vi "DIAdem Request Query.vi"(5 "Logic String":string, 6 "result columns (comma list)":string, 7 "Conditions String":string, 8 "error in (no error)":errorcluster, 9 "Username (empty)":string, 10 "Query Name":string="Spartan_Query.VBS", 11 "Query TDM":path) -> (0 "error out":errorcluster, 2 "Timed Out?":bool, 3 "Result":string)   [LabVIEW 2011]
uses:
  DIAdem Daemon Queue.ctl
  DIAdem Daemon Script Type.ctl
  Addons/internet/utils/strutil.llb/Case Matching.ctl
  server lib/Spartan CONFIG Global.vi
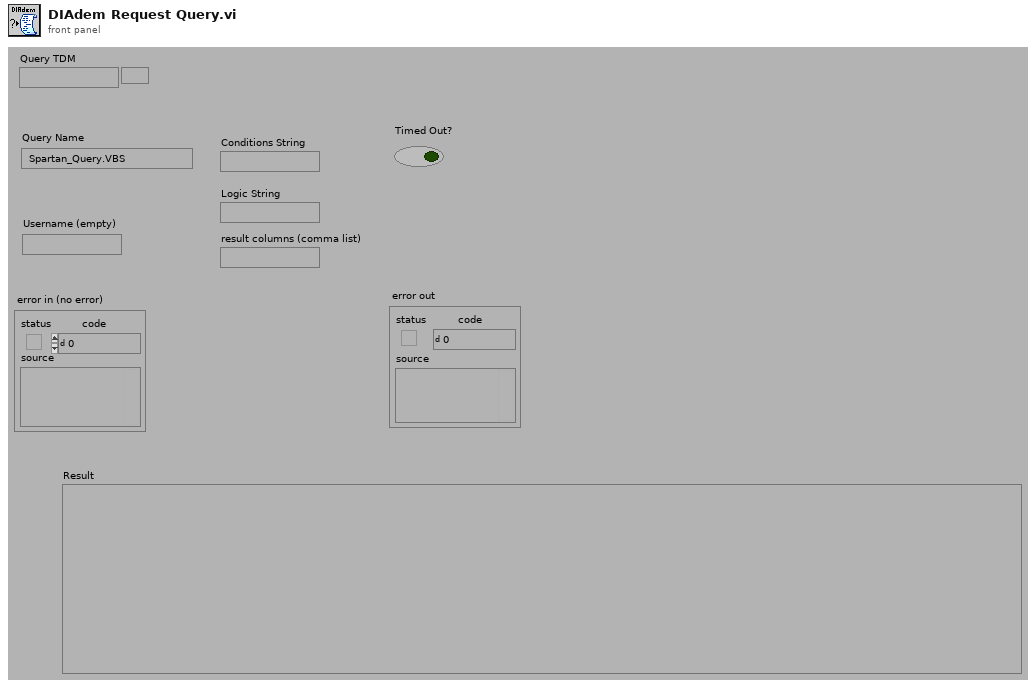
[diagram p1: front panel]
types:
  T1 = typedef "Case Matching.ctl" = enum16{"a != A", "a == A", "system"}
  T2 = typedef "DIAdem Daemon Script Type.ctl" = enum16{"Report", "Query", "Script", "Datasheet", "Append", "Restart", "Stop"}
  T3 = typedef "DIAdem Daemon Queue.ctl" = cluster{"Report Template TDM":path, "Report Processor VBS":path, "Report Path PDF":path, "Report Script Params":string, "Username":string, "Script Type":T2, "Report Query Params":string, "Client Machine":string, "Print on Client?":bool, "Response Queue Name":string, "Script Variables":string[], "Start Request Time":timestamp, "Wait?":bool}
  T4 = typedef "Keyed Array.ctl" = cluster{"keys":string[], "values":string[]}
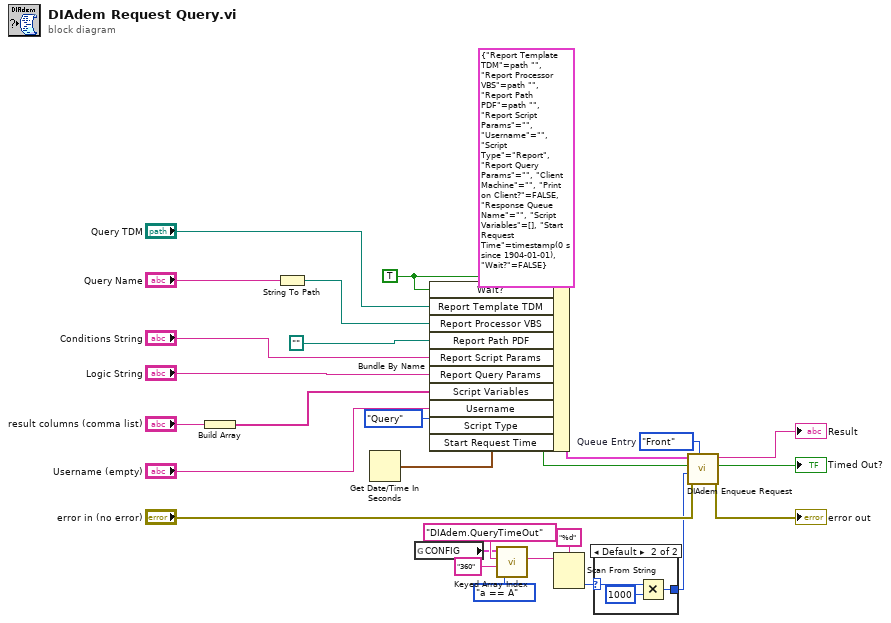
[diagram p0: block diagram]
diagram:
  w12 = enum16{"Front", "Back"}."Front"  # Queue Entry
  w9 = TRUE ("Wait for Completion?")
  n1 = Build Array("result columns (comma list)") -> (w10:string[])
  n2 = String To Path(string="Query Name") -> (path=w21:path)
  n3 = Get Date/Time In Seconds() -> (seconds since 1Jan1904=w14:timestamp)
  n4 = global read "Spartan CONFIG Global.vi" "CONFIG"() -> (w5:T4)
  n5 = Bundle By Name(cluster=T3 {"Report Template TDM"=path "", "Report Processor VBS"=path "", "Report Path PDF"=path "", "Report Script Params"="", "Username"="", "Script Type"=enum."Report", "Report Query Params"="", "Client Machine"="", "Print on Client?"=FALSE, "Response Queue Name"="", "Script Variables"=[], "Start Request Time"=timestamp(0 s since 1904-01-01), "Wait?"=FALSE} ("DD_Report"), "Wait?"=w9, "Report Template TDM"="Query TDM", "Report Processor VBS"=w21, "Report Path PDF"=path "", "Report Script Params"="Conditions String", "Report Query Params"="Logic String", "Script Variables"=w10, "Username"="Username (empty)", "Script Type"=DIAdem_Daemon_Script_Type."Query", "Start Request Time"=w14) -> (w18:T3)
  n6 = call "Keyed Array Index.vi"("case matching (sensitive)"=Case_Matching."a == A", "default value"="360", "key"="DIAdem.QueryTimeOut", "array in"=w5) -> ("value"=w3:string)  [unwired: 3 out]
  n7 = Scan From String(format string="%d" ("regular expression"), input string=w3) -> (output 1=w2:i32)  [unwired: 3 in, 3 out]
  n8 = case shown="Default" w2 {
    selector: w2 -> [w28 w30]
    tunnel: [w28 w29] -> w1
    frame -1 {
      # "No Timeout"
    }
    frame Default {
      n9 = Multiply(x=w30, y=1000) -> (x*y=w29:i32)
    }
  }
  n10 = call "DIAdem Enqueue Request.vi"("Queue Entry"=w12, "error in (no error)"="error in (no error)", "timeout in ms (300000)"=w1, "Wait for Completion? (f)"=w9, "DD_Report"=w18) -> ("error out"=→"error out":errorcluster, "timed out?"=→"Timed Out?":bool, "Results"=→"Result":string)  [unwired: 4 out]
